vi "(Depricated) Handle Idle.vi"(8 "error in (no error)":errorcluster, 11 "cRIO-CO2 in":refnum<class "cRIO-CO2.lvclass">=refnum) -> (0 "error out":errorcluster, 2 "cRIO-CO2 State":T1, 3 "cRIO-CO2 out":refnum<class "cRIO-CO2.lvclass">)   [LabVIEW 2015]
uses:
  cRIO-CO2.lvclass
  State Enumerator.ctl
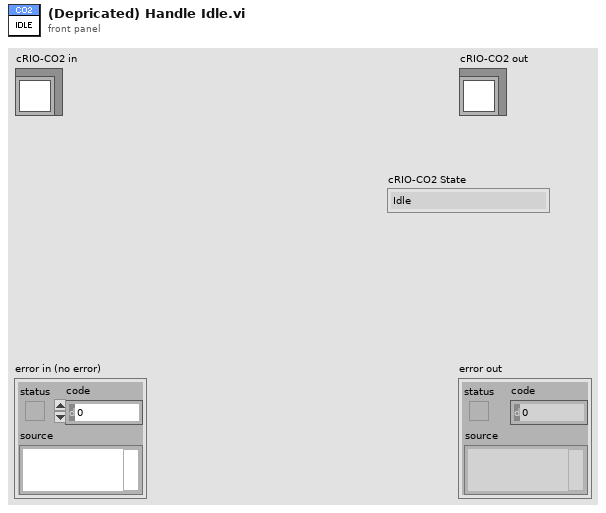
[diagram p1: front panel]
types:
  T1 = typedef "State Enumerator.ctl" = enum16{"Idle", "Initialize"}
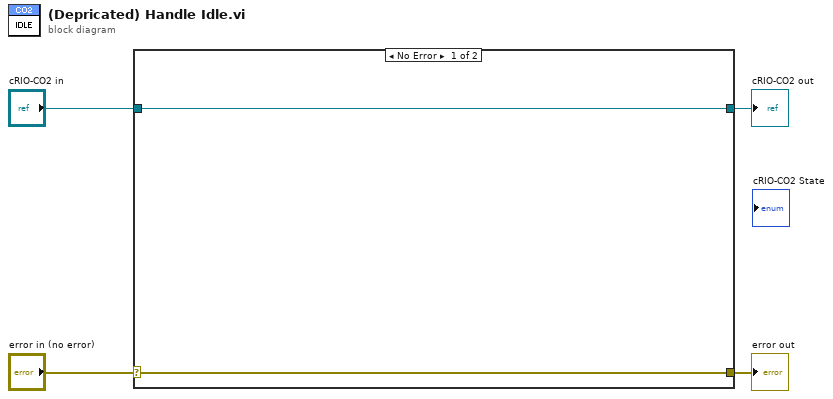
[diagram p0: block diagram]
diagram:
  n1 = case shown="No Error" "error in (no error)" {
    selector: "error in (no error)" -> [w5 w8]
    tunnel: [w5 w8] -> w3
    tunnel: [w6 w7] -> w1
    tunnel: "cRIO-CO2 in" -> [w6 w7]
    frame No Error {
    }
    frame Error {
    }
  }
  "error out" <- w3
  "cRIO-CO2 out" <- w1
